vi "HIOKI PW3390 Initialize RS-232C.vi"(0 "COM Port":refnum<visa-resource-name>="COM1", 1 "ID Query (T: Yes)":bool=TRUE, 2 "Reset (F: No)":bool, 5 "baud rate (38400bps)":u32=38400, 11 "error in (no error)":errorcluster) -> (4 "VISA Resource out":refnum<visa-resource-name>, 6 "ID":string, 15 "error out":errorcluster)   [LabVIEW 2018]
doc: "Starts the communication with the PW3390 device. This instance can select from the \"HIOKI PW3390 Initialize.vi (Polymorphic VI)\"."
uses:
  <vilib>/Instr/_visa.llb/VISA Configure Serial Port (Instr).vi
  <vilib>/Instr/_visa.llb/VISA Open Access Mode.ctl
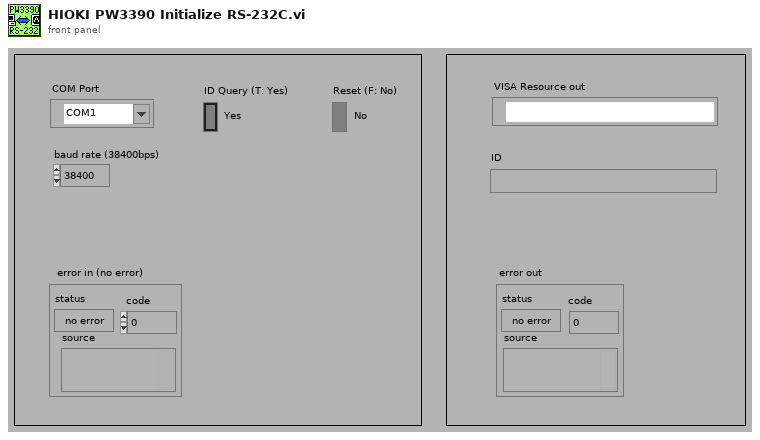
[diagram p1: front panel]
types:
  T1 = typedef "VISA Open Access Mode.ctl" = u32
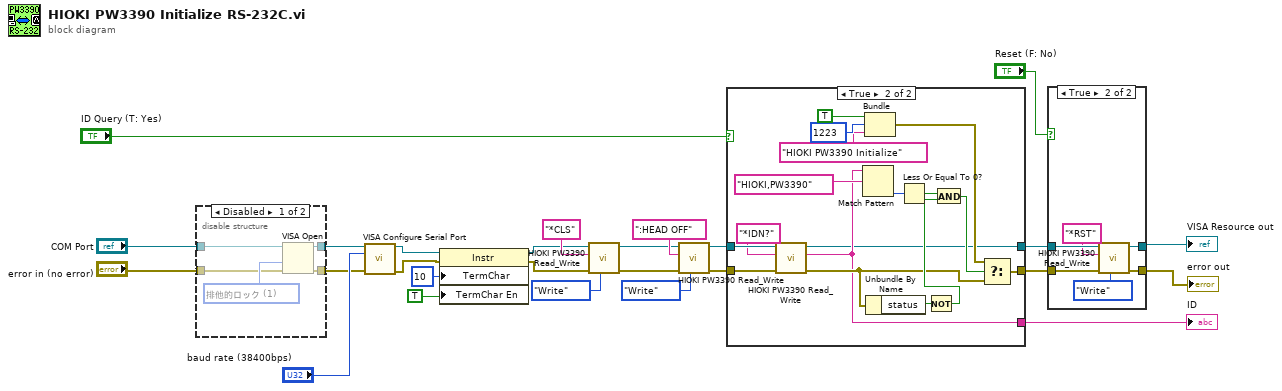
[diagram p0: block diagram]
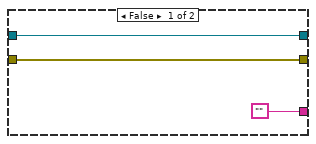
[diagram p4: hidden frame]
diagram:
  n1 = disable-structure shown="Disabled" {
    disable-tunnel: [w30 w33] -> w4
    disable-tunnel: "COM Port" -> [w29 w33]
    disable-tunnel: "error in (no error)" -> [w28 w32]
    disable-tunnel: [w27 w32] -> w1
    frame Disabled {
      w31 = T1 1 items=["VISAデフォルト"=0, "排他的ロック"=1, "構成設定をロード"=4] ("Access Mode")
      n2 = VISA Open(access mode=w31, error in (no error)=w28, VISA resource name=w29) -> (VISA resource name=w30:refnum<visa-resource-name>, error out=w27:errorcluster)  [unwired: 2 in]
    }
    frame Enabled {
    }
  }
  n3 = call-poly "VISA Configure Serial Port"("VISA resource name"=w4, "baud rate (9600)"="baud rate (38400bps)", "error in (no error)"=w1) -> ("VISA resource name out"=w7:refnum<visa-resource-name>, "error out"=w6:errorcluster)  [unwired: 11 in]
  n4 = property class="Instr"(reference=w7, error in=w6, "TermChar"=u8 10 ("Message Based Settings:Termination Character"), "TermChar En"=TRUE ("Message Based Settings:Termination Character Enable")) -> (reference out=w9:refnum<visa-resource-name>, error out=w8:errorcluster)
  n5 = call "HIOKI PW3390 Read_Write.vi"("Read/Write"=enum16{"Read", "Write"}."Write", "error in (no error)"=w8, "data in"="*CLS", "VISA Resource"=w9) -> ("error out"=w13:errorcluster, "VISA Resource out"=w14:refnum<visa-resource-name>)  [unwired: 5 in, 1 out]
  n6 = call "HIOKI PW3390 Read_Write.vi"("Read/Write"=enum16{"Read", "Write"}."Write", "error in (no error)"=w13, "data in"=":HEAD OFF", "VISA Resource"=w14) -> ("error out"=w19:errorcluster, "VISA Resource out"=w18:refnum<visa-resource-name>)  [unwired: 5 in, 1 out]
  n7 = case shown="True" "ID Query (T: Yes)" {
    tunnel: w19 -> [w35 w41]
    tunnel: [w35 w49] -> w25
    tunnel: w18 -> [w36 w42]
    tunnel: [w36 w37] -> w26
    tunnel: ["" ("読み込みﾊﾞｯﾌｧ") w38] -> w23
    frame False {
    }
    frame True {
      n8 = call "HIOKI PW3390 Read_Write.vi"("error in (no error)"=w41, "data in"="*IDN?", "VISA Resource"=w42) -> ("error out"=w40:errorcluster, "data out"=w38:string, "VISA Resource out"=w37:refnum<visa-resource-name>)  [unwired: 6 in]
      n9 = Match Pattern(string=w38, regular expression="HIOKI,PW3390") -> (offset past match=w52:i32)  [unwired: 1 in, 3 out]
      n10 = Bundle("status"=TRUE, "code"=1223, "source"="HIOKI PW3390 Initialize") -> (w48:errorcluster)  [unwired: 1 in]
      n11 = Unbundle By Name(w40) -> ("status"=w44:bool)
      n12 = Less Or Equal To 0?(x=w52) -> (x <= 0?=w51:bool)
      n13 = Not(x=w44) -> (.not. x?=w43:bool)
      n14 = And(x=w51, y=w43) -> (x .and. y?=w50:bool)
      n15 = Select(t=w48, s=w50, f=w40) -> (s? t:f=w49:errorcluster)
    }
  }
  "ID" <- w23
  n16 = case shown="True" "Reset (F: No)" {
    tunnel: w26 -> [w54 w61]
    tunnel: w25 -> [w55 w60]
    tunnel: [w55 w59] -> w24
    tunnel: [w54 w56] -> w12
    frame False {
    }
    frame True {
      n17 = call "HIOKI PW3390 Read_Write.vi"("Read/Write"=enum16{"Read", "Write"}."Write", "error in (no error)"=w60, "data in"="*RST", "VISA Resource"=w61) -> ("error out"=w59:errorcluster, "VISA Resource out"=w56:refnum<visa-resource-name>)  [unwired: 5 in, 1 out]
    }
  }
  "error out" <- w24
  "VISA Resource out" <- w12
